vi "GlobalDriverStationCommands.vi"() -> ()   [LabVIEW 2020]
doc: "This global variable contains driver, manipulator, and autonomous command instructions. The variables here must be maintained such that they cannot change when the robot is disabled unless super-test mode is enabled."
panel:
  out "Manipulator_RightTrigger":dbl
  out "Manipulator_RightY":dbl
  out "Manipulator_RightX":dbl
  out "Manipulator_LeftX":dbl
  out "Manipulator_LeftTrigger":dbl
  out "Manipulator_LeftY":dbl
  out "Manipulator_RightTriggerBoolean":bool
  out "Manipulator_LeftTriggerBoolean":bool
  out "Manipulator_LeftJoystickButton":bool
  out "Manipulator_RightJoystickButton":bool
  out "Manipulator_RightBumper":bool
  out "Manipulator_LeftBumper":bool
  out "Manipulator_Menu":bool
  out "Manipulator_View":bool
  out "Manipulator_Y":bool
  out "Manipulator_X":bool
  out "Manipulator_B":bool
  out "Manipulator_A":bool
  out "Driver_RightTrigger":dbl
  out "Driver_RightY":dbl
  out "Driver_RightX":dbl
  out "Driver_LeftX":dbl
  out "Driver_LeftTrigger":dbl
  out "Driver_LeftY":dbl
  out "Driver_RightTriggerBoolean":bool
  out "Driver_LeftTriggerBoolean":bool
  out "Driver_LeftJoystickButton":bool
  out "Driver_RightJoystickButton":bool
  out "Driver_RightBumper":bool
  out "Driver_LeftBumper":bool
  out "Driver_Menu":bool
  out "Driver_View":bool
  out "Driver_Y":bool
  out "Driver_X":bool
  out "Driver_B":bool
  out "Driver_A":bool
  # "DRIVER JOYSTICK"
  # "MANIPULATOR JOYSTICK"
  # "AUTONOMOUS ONLY"
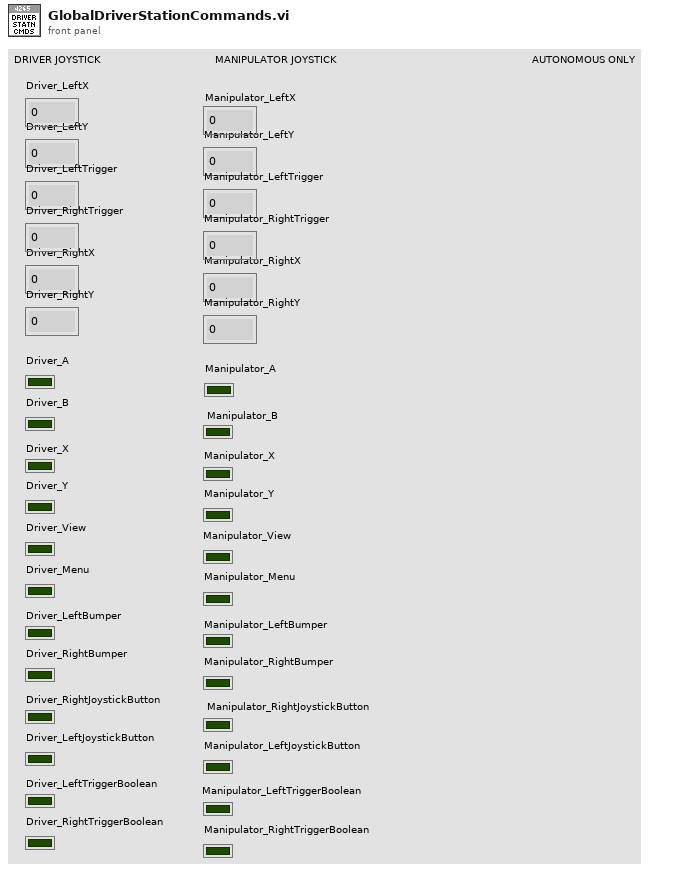
[diagram p1: front panel]
diagram:
